vi "Mcp2210 Cancel Spi Txfer.vi"(8 "error in (no error)":errorcluster, 11 "handle":i32) -> (0 "error out":errorcluster, 1 "SPI Current Owner":enum16{"No Owner", "USB Bridge", "Ext. Master"}(ring), 2 "SPI Release Ext Req Status":T1(ring), 3 "handle out":i32)   [LabVIEW 2015, in "mcp2210.lvlib"]
doc: "Cancel the current SPI transfer and provides information about:\n- SPI Bus release external request status,\n- SPI Bus ownership prior the command (who is the Master).\nThe command also releases the bus ownership.\nParameters:\nInputs:\n- void *handle - The pointer to the device handle. Cannot be NULL.\nOutputs:\n- unsigned char *pspiExtReqStat - SPI Bus release external request status:\n- 0x01 ¨C No External Request for SPI Bus Release\n- 0x00 ¨C Pending External Request for SPI Bus Release\nCannot be NULL.\n- unsigned char *pspiOwner - SPI Bus current owner:\n- 0x00 - No owner\n- 0x01 - USB Bridge\n- 0x02 - External Master.\nCannot be NULL.\nReturns:\n- 0 for success: E_SUCCESS\n- negative error code: E_ERR_NULL, E_ERR_INVALID_HANDLE_VALUE\nE_ERR_UNKOWN_ERROR\nE_ERR_HID_TIMEOUT, E_ERR_HID_RW_FILEIO\nE_ERR_CMD_ECHO, E_ERR_CMD_FAILED\n\nMCP2210_DLL_UM_API int __stdcall Mcp2210_CancelSpiTxfer(void *handle, unsigned char *pspiExtReqStat, unsigned char *pspiOwner);"
uses:
  <userlib>/mcp2210/mcp2210.lvlib
  <userlib>/mcp2210/mcp2210_dll_um_x86.dll
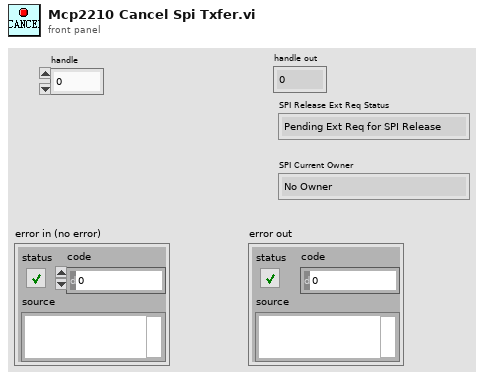
[diagram p1: front panel]
types:
  T1 = enum16{"Pending Ext Req for SPI Release", "No Ext Req for SPI Release"}
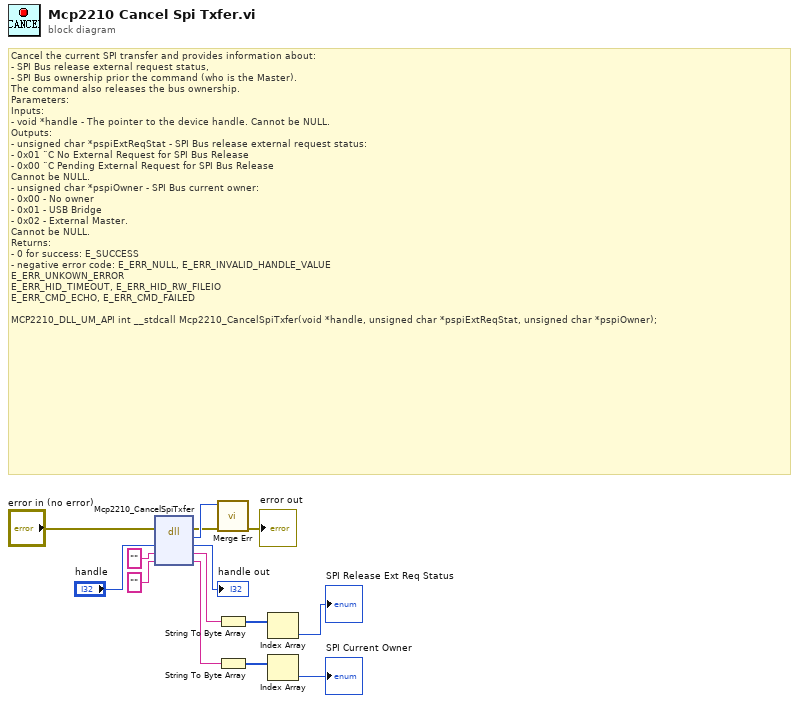
[diagram p0: block diagram]
diagram:
  # "Cancel the current SPI transfer and provides information about:\n- SPI Bus release external request status,\n- SPI Bus ownership prior the command (who is the Master).\nThe command also releases the bus ownership.\nParameters:\nInputs:\n- void *handle - The pointer to the device handle. Cannot be NULL.\nOutputs:\n- unsigned char *pspiExtReqStat - SPI Bus release external request status:\n- 0x01 ¨C No External Request for SPI Bus Release\n- 0x00 ¨C Pending External Request for SPI Bus Release\nCannot be NULL.\n- unsigned char *pspiOwner - SPI Bus current owner:\n- 0x00 - No owner\n- 0x01 - USB Bridge\n- 0x02 - External Master.\nCannot be NULL.\nReturns:\n- 0 for success: E_SUCCESS\n- negative error code: E_ERR_NULL, E_ERR_INVALID_HANDLE_VALUE\nE_ERR_UNKOWN_ERROR\nE_ERR_HID_TIMEOUT, E_ERR_HID_RW_FILEIO\nE_ERR_CMD_ECHO, E_ERR_CMD_FAILED\n\nMCP2210_DLL_UM_API int __stdcall Mcp2210_CancelSpiTxfer(void *handle, unsigned char *pspiExtReqStat, unsigned char *pspiOwner);"
  n1 = dll-call lib="D:/LabVIEW 2015/user.lib/mcp2210/mcp2210_dll_um_x86.*" fn="Mcp2210_CancelSpiTxfer"(error in="error in (no error)", "handle"="handle", "pspiExtReqStat"="", "pspiOwner"="") -> (error out=w9:errorcluster, "return type"=w10:i32, "handle"=→"handle out":u32, "pspiExtReqStat"=w6:string, "pspiOwner"=w3:string)  [unwired: 2 in, 1 out]
  n2 = call <userlib>:"Merge Err.vi"("error in (no error)"=w9, "return type"=w10) -> ("error out"=→"error out":errorcluster)  [unwired: 9 in]
  n3 = String To Byte Array(string=w6) -> (unsigned byte array=w5:u8[])
  n4 = String To Byte Array(string=w3) -> (unsigned byte array=w2:u8[])
  n5 = Index Array(array=w5) -> (element=→"SPI Release Ext Req Status":u8)  [unwired: 1 in]
  n6 = Index Array(array=w2) -> (element=→"SPI Current Owner":u8)  [unwired: 1 in]
